vi "Test.vi"   [LabVIEW 2018]
doc: "This VI is called when test mode begins, and will automatically be terminated when it ends. You can add manual or automatic tests and invoke them from the dashboard."
uses:
  SubVis/Test Mode/Test Mode Global.vi
types:
  T1 = cluster{"Drive Test?":bool, "Cargo Test?":bool, "Hatch Test?":bool, "Lift Test?":bool}
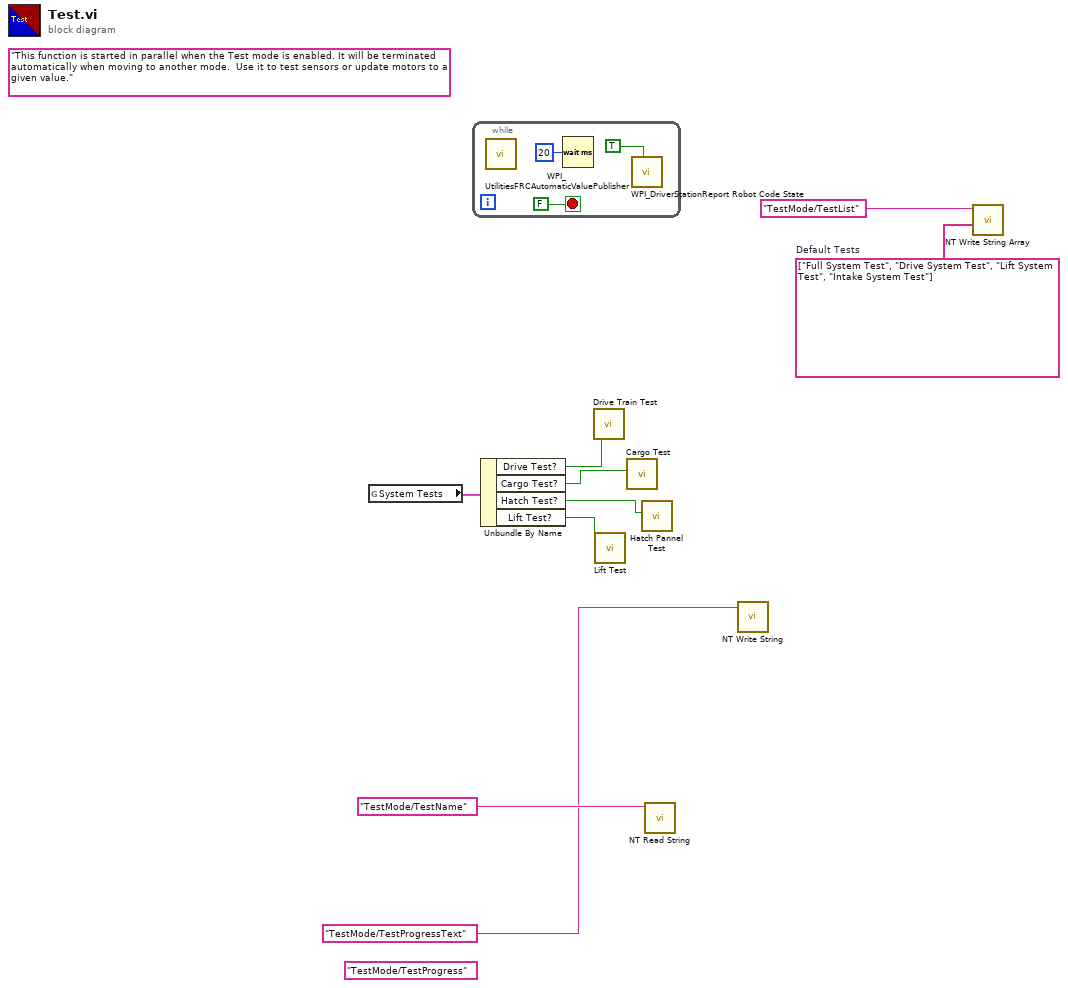
[diagram p0: block diagram]
diagram:
  w7 = string[] ["Full System Test", "Drive System Test", "Lift System Test", "Intake System Test"]  # Default Tests
  (unwired) "TestMode/TestProgress" ("Name")
  (unwired) "This function is started in parallel when the Test mode is enabled. It will be terminated automatically when moving to another mode.  Use it to test sensors or update motors to a given value."
  n1 = global read "Test Mode Global.vi" "System Tests"() -> (w5:T1)
  n2 = while {
    stop <- FALSE stop-if-true
    n3 = call <vilib>:"WPI_UtilitiesFRCAutomaticValuePublisher.vi"() -> ()  [unwired: 12 in]
    n4 = Wait (ms)(milliseconds to wait=u32 20) -> ()  [unwired: 1 out]
    n5 = call <vilib>:"WPI_DriverStationReport Robot Code State.vi"("Test"=TRUE ("Autonomous")) -> ()  [unwired: 10 in, 1 out]
  }
  n6 = Unbundle By Name(w5) -> ("Drive Test?"=w4:bool, "Cargo Test?"=w2:bool, "Hatch Test?"=w1:bool, "Lift Test?"=w3:bool)
  n7 = call "Drive Train Test.vi"("Boolean"=w4) -> ()  [unwired: 11 in]
  n8 = call "Lift Test.vi"("Run?"=w3) -> ()  [unwired: 11 in]
  n9 = call "Cargo Test.vi"("Run"=w2) -> ()  [unwired: 11 in]
  n10 = call "Hatch Pannel Test.vi"("Run?"=w1) -> ()  [unwired: 11 in]
  n11 = call <vilib>:"NT Read String.vi"("Name"="TestMode/TestName") -> ()  [unwired: 9 in, 2 out]
  n12 = call <vilib>:"NT Write String.vi"("Name"="TestMode/TestProgressText") -> ()  [unwired: 10 in, 1 out]
  n13 = call <vilib>:"NT Write String Array.vi"("String Array"=w7, "Name"="TestMode/TestList") -> ()  [unwired: 9 in, 1 out]
